vi "Robot Global Data.vi"() -> ()   [LabVIEW 2011]
doc: "This global VI can contain as many global variables as you need. Place a control on the panel, give it a good name. To read or write to it from a VI, drag the icon to the diagram of that VI. You can also drag from the project. Click on the node to change which global you access. You shouldn't have multiple locations writing to a global or it will cause a race-condition."
uses:
  <vilib>/Rock Robotics/WPI/Camera/WPI_CameraImageSize.ctl
  Shared/cRIO Performance Details.ctl
  Shared/Drive Base Dashboard Package.ctl
  Shared/Shifter State.ctl
  Apendage State.ctl
panel:
  in  "Horn Switch":bool
  in  "Horn":T1=enum."Up"
  in  "Arm":T1=enum."Up"
  out "Drive Base":T2
  in  "Performance Details":T4 {"CPU Utilization" format="%#.2f"}
  in  "LED toggle rate (ms)":u32=20
  in  "image size":T5=enum."320x240"
  in  "Enable Vision":bool
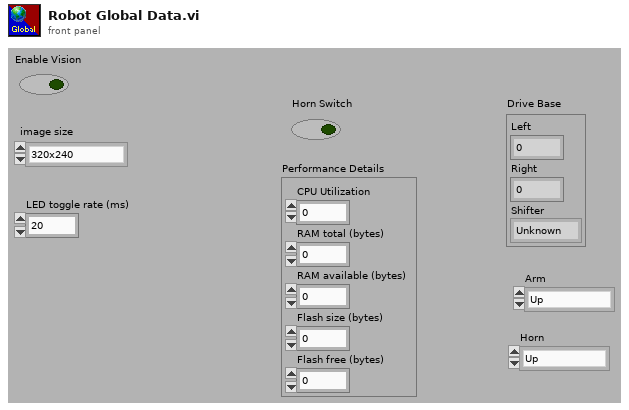
[diagram p1: front panel]
types:
  T1 = typedef "Apendage State.ctl" = enum16{"Unknown", "Down", "Up"}
  T2 = typedef "Drive Base Dashboard Package.ctl" = cluster{"Left":dbl, "Right":dbl, "Shifter":T3}
  T3 = typedef "Shifter State.ctl" = enum16{"Unknown", "Low", "High"}
  T4 = typedef "cRIO Performance Details.ctl" = cluster{"CPU Utilization":dbl, "RAM total (bytes)":u32, "RAM available (bytes)":u32, "Flash size (bytes)":i64, "Flash free (bytes)":i64}
  T5 = typedef "WPI_CameraImageSize.ctl" = enum16{"640x480", "320x240", "160x120"}
diagram:
